vi "WRO_BB Main.vi"() -> ()   [LabVIEW 2014]
uses:
  <vilib>/myRIO/Common/Instrument Driver Framework/myRIO v1.0/UART/vis/myRIO v1.0 Close UART.vi
  <vilib>/myRIO/Common/Instrument Driver Framework/Utilities/vis/FPGA Ref Manager.vi
  <vilib>/myRIO/Common/Instrument Driver Framework/myRIO v1.0/myRIO v1.0 Reset FPGA.vi
  <vilib>/myRIO/Common/Instrument Driver Framework/myRIO v1.0/IRQ/vis/myRIO v1.0 IRQ Info FGV.vi
  <vilib>/myRIO/Common/Instrument Driver Framework/myRIO v1.0/IRQ/vis/myRIO v1.0 Timer IRQ Info FGV.vi
  <vilib>/myRIO/Common/Instrument Driver Framework/myRIO v1.0/IRQ/vis/myRIO v1.0 ISR Agent.vi
  <vilib>/myRIO/Instrument Drivers/Utilities/Utilities.lvlib
panel:
  out "error out":errorcluster
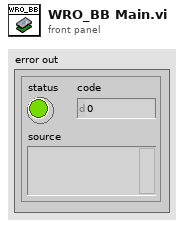
[diagram p1: front panel]
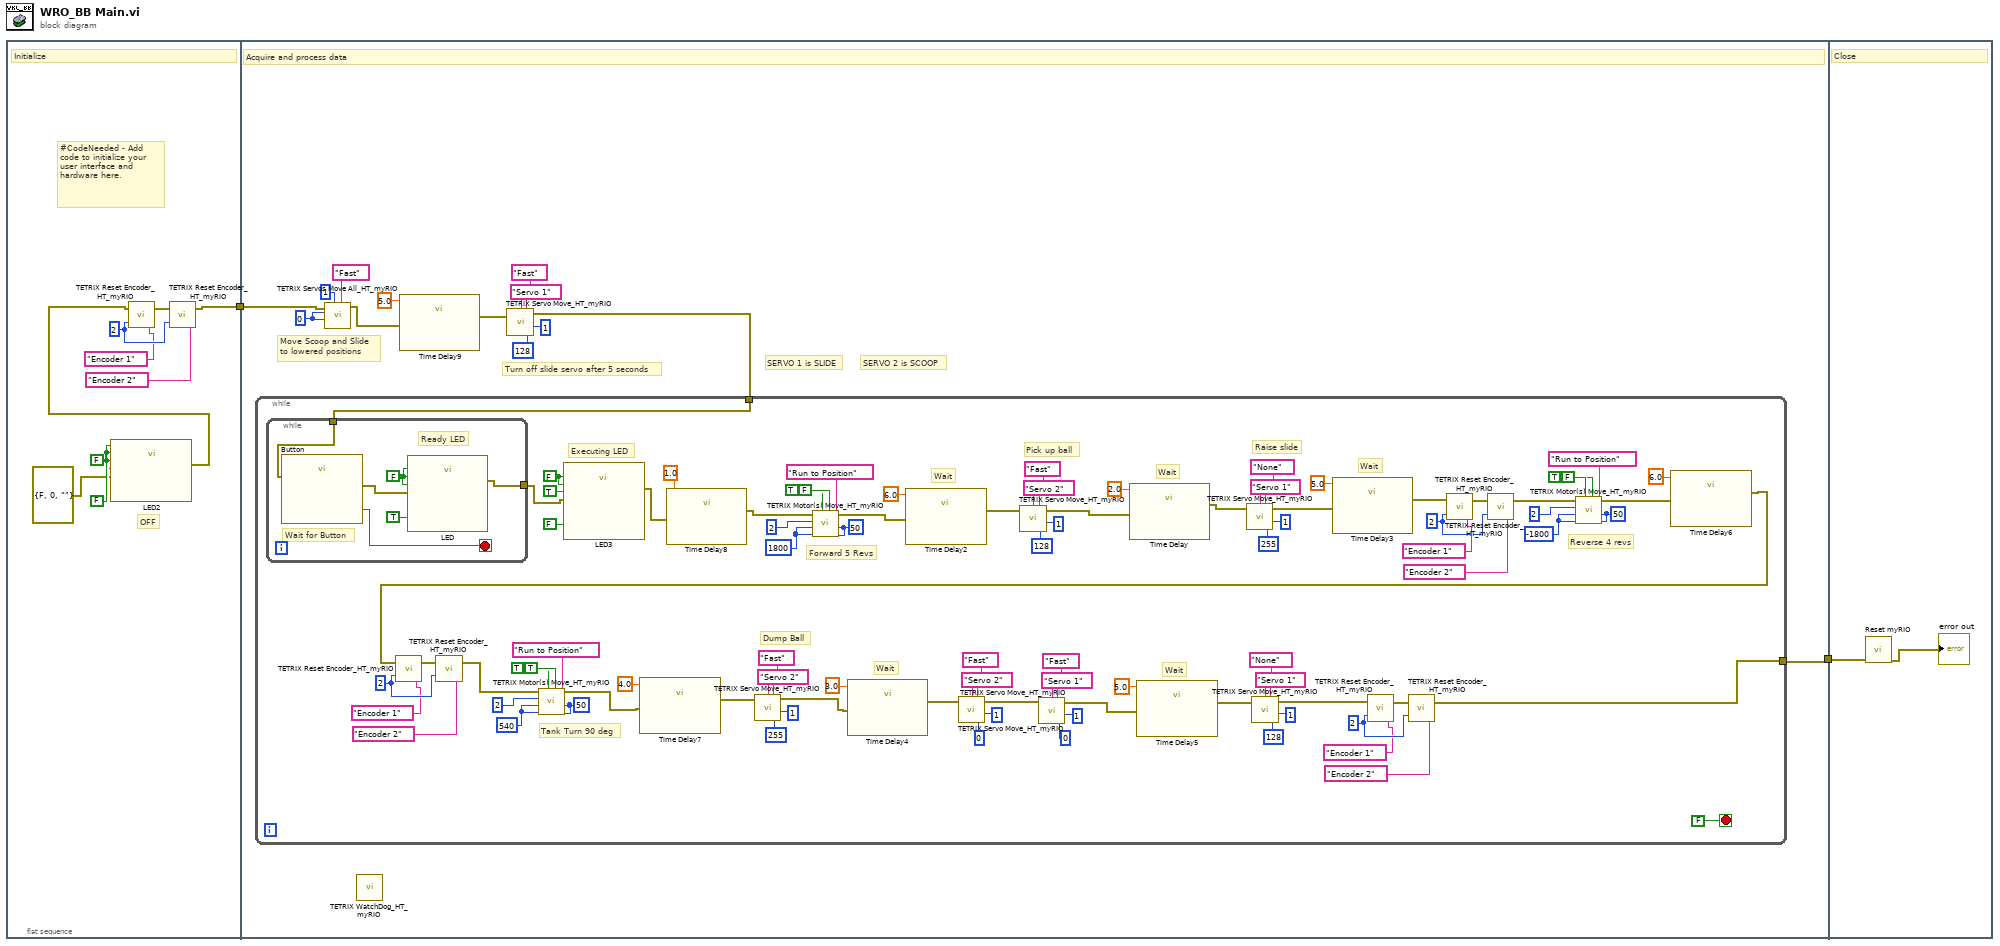
[diagram p0: block diagram]
diagram:
  n1 = flat-sequence {
    tunnel: [w7] -> w2
    tunnel: w2 -> [w13]
    tunnel: [w12] -> w1
    tunnel: w1 -> [w121]
    frame #0 {
      w3 = FALSE ("LED2")
      w11 = u8 2 ("Controller Daisy Chain Position ( 1 - 4)")
      # "OFF"
      # "#CodeNeeded - Add code to initialize your user interface and hardware here."
      # "Initialize"
      n2 = call "LED2"("Ready"=FALSE, "LED1"=w3, "LED2"=w3, "LED3"=w3, "error in (no error)"=errorcluster {"status"=FALSE, "code"=0, "source"=""} ("error out")) -> ("error out"=w4:errorcluster)  [unwired: 22 in]
      n3 = call "TETRIX Reset Encoder_HT_myRIO.vi"("Select Encoder"="Encoder 1", "Controller Daisy Chain Position ( 1 - 4)"=w11, "error in (no error)"=w4) -> ("error out"=w8:errorcluster)
      n4 = call "TETRIX Reset Encoder_HT_myRIO.vi"("Select Encoder"="Encoder 2", "Controller Daisy Chain Position ( 1 - 4)"=w11, "error in (no error)"=w8) -> ("error out"=w7:errorcluster)
    }
    frame #1 {
      w24 = u8 0 ("Servo 1 (0 - 255)")
      # "Turn off slide servo after 5 seconds"
      # "Move Scoop and Slide\nto lowered positions"
      # "SERVO 1 is SLIDE"
      # "SERVO 2 is SCOOP"
      # "Acquire and process data"
      n5 = call "TETRIX Servos Move All_HT_myRIO.vi"("Enable Sync: Fast | Medium | Slow | None"="Fast", "Controller Daisy Chain Position (1 - 4)"=u8 1, "Servo 2 (0 - 255)"=w24, "Servo 1 (0 - 255)"=w24, "error in (no error)"=w13) -> ("error out"=w16:errorcluster)  [unwired: 4 in]
      n6 = call "TETRIX WatchDog_HT_myRIO.vi"() -> ()  [unwired: 3 in, 1 out]
      n7 = call "Time Delay9"("error in (no error)"=w16, "Delay Time (s)"=5.0) -> ("error out"=w15:errorcluster)  [unwired: 9 in]
      n8 = call "TETRIX Servo Move_HT_myRIO.vi"("Servo Position (0 - 255)"=u8 128, "Controller Daisy Chain Position (1 - 4)"=u8 1, "Enable Sync: Fast | Medium | Slow | None"="Fast", "Select Servo"="Servo 1", "error in (no error)"=w15) -> ("error out"=w14:errorcluster)
      n9 = while {
        tunnel: w14 -> [w31]
        tunnel: [w30] -> w12
        stop <- FALSE stop-if-true
        w28 = FALSE ("LED1")
        w36 = u8 2 ("Controller Daisy Chain Position ( 1 - 4)")
        w63 = 540 ("Encoder Target (-2147483648 to 2147483647)\n1440 = 1 revolution")
        w65 = i8 50 ("Motor 1 Power (-100 to 100)\n0 = Stop/Brake\n-128 = Stop/Coast")
        w71 = u8 2 ("Controller Daisy Chain Position ( 1 - 4)")
        w77 = -1800 ("Encoder Target (-2147483648 to 2147483647)\n1440 = 1 revolution")
        w75 = i8 50 ("Motor 1 Power (-100 to 100)\n0 = Stop/Brake\n-128 = Stop/Coast")
        w101 = 1800 ("Encoder Target (-2147483648 to 2147483647)\n1440 = 1 revolution")
        w103 = i8 50 ("Motor 1 Power (-100 to 100)\n0 = Stop/Brake\n-128 = Stop/Coast")
        w81 = u8 2 ("Controller Daisy Chain Position ( 1 - 4)")
        # "Executing LED"
        # "Tank Turn 90 deg"
        # "Forward 5 Revs"
        # "Reverse 4 revs"
        # "Wait"
        # "Wait"
        # "Wait"
        # "Wait"
        # "Wait"
        # "Dump Ball"
        # "Raise slide"
        # "Pick up ball"
        n10 = while {
          tunnel: [w115] -> w26
          tunnel: w31 -> [w118]
          stop <- w119 stop-if-true
          w114 = FALSE ("LED2")
          # "Wait for Button"
          # "Ready LED"
          n11 = call "Button"("error in (no error)"=w118) -> ("Value"=w119:bool, "error out"=w117:errorcluster)  [unwired: 25 in]
          n12 = call "LED"("Ready"=TRUE, "LED1"=w114, "LED2"=w114, "LED3"=w114, "error in (no error)"=w117) -> ("error out"=w115:errorcluster)  [unwired: 22 in]
        }
        n13 = call "LED3"("Ready"=FALSE, "LED1"=w28, "LED2"=w28, "LED3"=TRUE, "error in (no error)"=w26) -> ("error out"=w25:errorcluster)  [unwired: 22 in]
        n14 = call "Time Delay8"("error in (no error)"=w25, "Delay Time (s)"=1.0) -> ("error out"=w98:errorcluster)  [unwired: 9 in]
        n15 = call "TETRIX Motor(s) Move_HT_myRIO.vi"("Motor 2 Power (-100 to 100)\n0 = Stop/Brake\n-128 = Stop/Coast"=w103, "Motor 1 Power (-100 to 100)\n0 = Stop/Brake\n-128 = Stop/Coast"=w103, "Control Mode"="Run to Position", "Motor 2 Reverse? : T or F"=FALSE, "Motor 1 Reverse? : T or F"=TRUE, "Encoder 2 Target: 360 = 1 motor shaft revolution"=w101, "Encoder 1 Target: 360 = 1 motor shaft revolution"=w101, "Controller Daisy Chain Position: 1 - 4"=u8 2, "error in (no error)"=w98) -> ("error out"=w97:errorcluster)
        n16 = call "Time Delay2"("error in (no error)"=w97, "Delay Time (s)"=6.0) -> ("error out"=w92:errorcluster)  [unwired: 9 in]
        n17 = call "TETRIX Servo Move_HT_myRIO.vi"("Servo Position (0 - 255)"=u8 128, "Controller Daisy Chain Position (1 - 4)"=u8 1, "Enable Sync: Fast | Medium | Slow | None"="Fast", "Select Servo"="Servo 2", "error in (no error)"=w92) -> ("error out"=w91:errorcluster)
        n18 = call "Time Delay"("error in (no error)"=w91, "Delay Time (s)"=2.0) -> ("error out"=w86:errorcluster)  [unwired: 9 in]
        n19 = call "TETRIX Servo Move_HT_myRIO.vi"("Servo Position (0 - 255)"=u8 255, "Controller Daisy Chain Position (1 - 4)"=u8 1, "Enable Sync: Fast | Medium | Slow | None"="None", "Select Servo"="Servo 1", "error in (no error)"=w86) -> ("error out"=w85:errorcluster)
        n20 = call "Time Delay3"("error in (no error)"=w85, "Delay Time (s)"=5.0) -> ("error out"=w80:errorcluster)  [unwired: 9 in]
        n21 = call "TETRIX Reset Encoder_HT_myRIO.vi"("Select Encoder"="Encoder 1", "Controller Daisy Chain Position ( 1 - 4)"=w81, "error in (no error)"=w80) -> ("error out"=w84:errorcluster)
        n22 = call "TETRIX Reset Encoder_HT_myRIO.vi"("Select Encoder"="Encoder 2", "Controller Daisy Chain Position ( 1 - 4)"=w81, "error in (no error)"=w84) -> ("error out"=w73:errorcluster)
        n23 = call "TETRIX Motor(s) Move_HT_myRIO.vi"("Motor 2 Power (-100 to 100)\n0 = Stop/Brake\n-128 = Stop/Coast"=w75, "Motor 1 Power (-100 to 100)\n0 = Stop/Brake\n-128 = Stop/Coast"=w75, "Control Mode"="Run to Position", "Motor 2 Reverse? : T or F"=FALSE, "Motor 1 Reverse? : T or F"=TRUE, "Encoder 2 Target: 360 = 1 motor shaft revolution"=w77, "Encoder 1 Target: 360 = 1 motor shaft revolution"=w77, "Controller Daisy Chain Position: 1 - 4"=u8 2, "error in (no error)"=w73) -> ("error out"=w72:errorcluster)
        n24 = call "Time Delay6"("error in (no error)"=w72, "Delay Time (s)"=6.0) -> ("error out"=w67:errorcluster)  [unwired: 9 in]
        n25 = call "TETRIX Reset Encoder_HT_myRIO.vi"("Select Encoder"="Encoder 1", "Controller Daisy Chain Position ( 1 - 4)"=w71, "error in (no error)"=w67) -> ("error out"=w68:errorcluster)
        n26 = call "TETRIX Reset Encoder_HT_myRIO.vi"("Select Encoder"="Encoder 2", "Controller Daisy Chain Position ( 1 - 4)"=w71, "error in (no error)"=w68) -> ("error out"=w60:errorcluster)
        n27 = call "TETRIX Motor(s) Move_HT_myRIO.vi"("Motor 2 Power (-100 to 100)\n0 = Stop/Brake\n-128 = Stop/Coast"=w65, "Motor 1 Power (-100 to 100)\n0 = Stop/Brake\n-128 = Stop/Coast"=w65, "Control Mode"="Run to Position", "Motor 2 Reverse? : T or F"=TRUE, "Motor 1 Reverse? : T or F"=TRUE, "Encoder 2 Target: 360 = 1 motor shaft revolution"=w63, "Encoder 1 Target: 360 = 1 motor shaft revolution"=w63, "Controller Daisy Chain Position: 1 - 4"=u8 2, "error in (no error)"=w60) -> ("error out"=w59:errorcluster)
        n28 = call "Time Delay7"("error in (no error)"=w59, "Delay Time (s)"=4.0) -> ("error out"=w54:errorcluster)  [unwired: 9 in]
        n29 = call "TETRIX Servo Move_HT_myRIO.vi"("Servo Position (0 - 255)"=u8 255, "Controller Daisy Chain Position (1 - 4)"=u8 1, "Enable Sync: Fast | Medium | Slow | None"="Fast", "Select Servo"="Servo 2", "error in (no error)"=w54) -> ("error out"=w53:errorcluster)
        n30 = call "Time Delay4"("error in (no error)"=w53, "Delay Time (s)"=3.0) -> ("error out"=w48:errorcluster)  [unwired: 9 in]
        n31 = call "TETRIX Servo Move_HT_myRIO.vi"("Servo Position (0 - 255)"=u8 0, "Controller Daisy Chain Position (1 - 4)"=u8 1, "Enable Sync: Fast | Medium | Slow | None"="Fast", "Select Servo"="Servo 2", "error in (no error)"=w48) -> ("error out"=w43:errorcluster)
        n32 = call "TETRIX Servo Move_HT_myRIO.vi"("Servo Position (0 - 255)"=u8 0, "Controller Daisy Chain Position (1 - 4)"=u8 1, "Enable Sync: Fast | Medium | Slow | None"="Fast", "Select Servo"="Servo 1", "error in (no error)"=w43) -> ("error out"=w42:errorcluster)
        n33 = call "Time Delay5"("error in (no error)"=w42, "Delay Time (s)"=5.0) -> ("error out"=w37:errorcluster)  [unwired: 9 in]
        n34 = call "TETRIX Servo Move_HT_myRIO.vi"("Servo Position (0 - 255)"=u8 128, "Controller Daisy Chain Position (1 - 4)"=u8 1, "Enable Sync: Fast | Medium | Slow | None"="None", "Select Servo"="Servo 1", "error in (no error)"=w37) -> ("error out"=w32:errorcluster)
        n35 = call "TETRIX Reset Encoder_HT_myRIO.vi"("Select Encoder"="Encoder 1", "Controller Daisy Chain Position ( 1 - 4)"=w36, "error in (no error)"=w32) -> ("error out"=w33:errorcluster)
        n36 = call "TETRIX Reset Encoder_HT_myRIO.vi"("Select Encoder"="Encoder 2", "Controller Daisy Chain Position ( 1 - 4)"=w36, "error in (no error)"=w33) -> ("error out"=w30:errorcluster)
      }
    }
    frame #2 {
      # "Close"
      n37 = call <vilib>:"Reset myRIO.vi"("error in (no error)"=w121) -> ("error out"=→"error out":errorcluster)  [unwired: 10 in]
    }
  }
